vi "build group channel lists.vi"() -> ()   [LabVIEW 2018]
uses:
  <userlib>/_OpenG.lib/array/array.llb/Filter 1D Array (DBL)__ogtk.vi
  <userlib>/_OpenG.lib/array/array.llb/Remove Duplicates from 1D Array (DBL)__ogtk.vi
panel:
  out "negative card groups":T1(array[cluster])
  out "ACTIVE":dbl[](array[numeric])
  out "Groups":T1(array[cluster])
  out "Empty groups":T1(array[cluster])
  out "GROUP00":dbl[](array[numeric])
  out "TANK":dbl[](array[numeric])
  out "MRD":dbl[](array[numeric])
  out "VETO":dbl[](array[numeric])
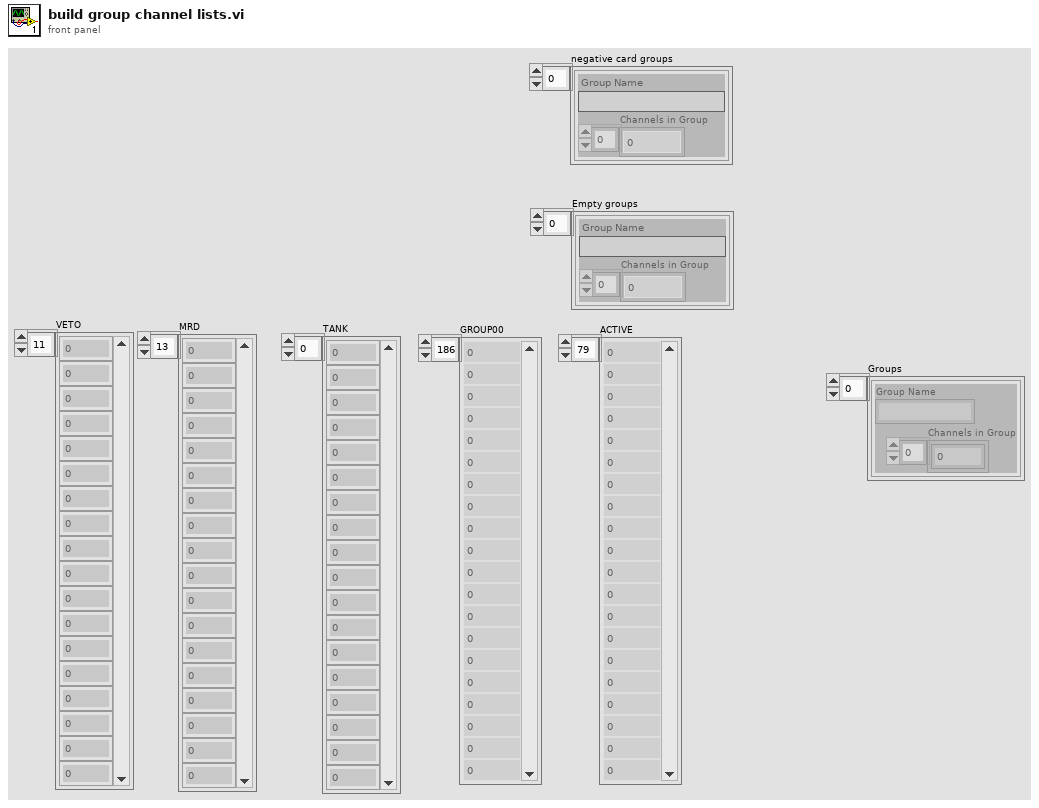
[diagram p1: front panel]
types:
  T1 = cluster{"Group Name":string, "Channels in Group":dbl[]}[]
  T2 = cluster{"Group Name":string, "Channels in Group":dbl[]}
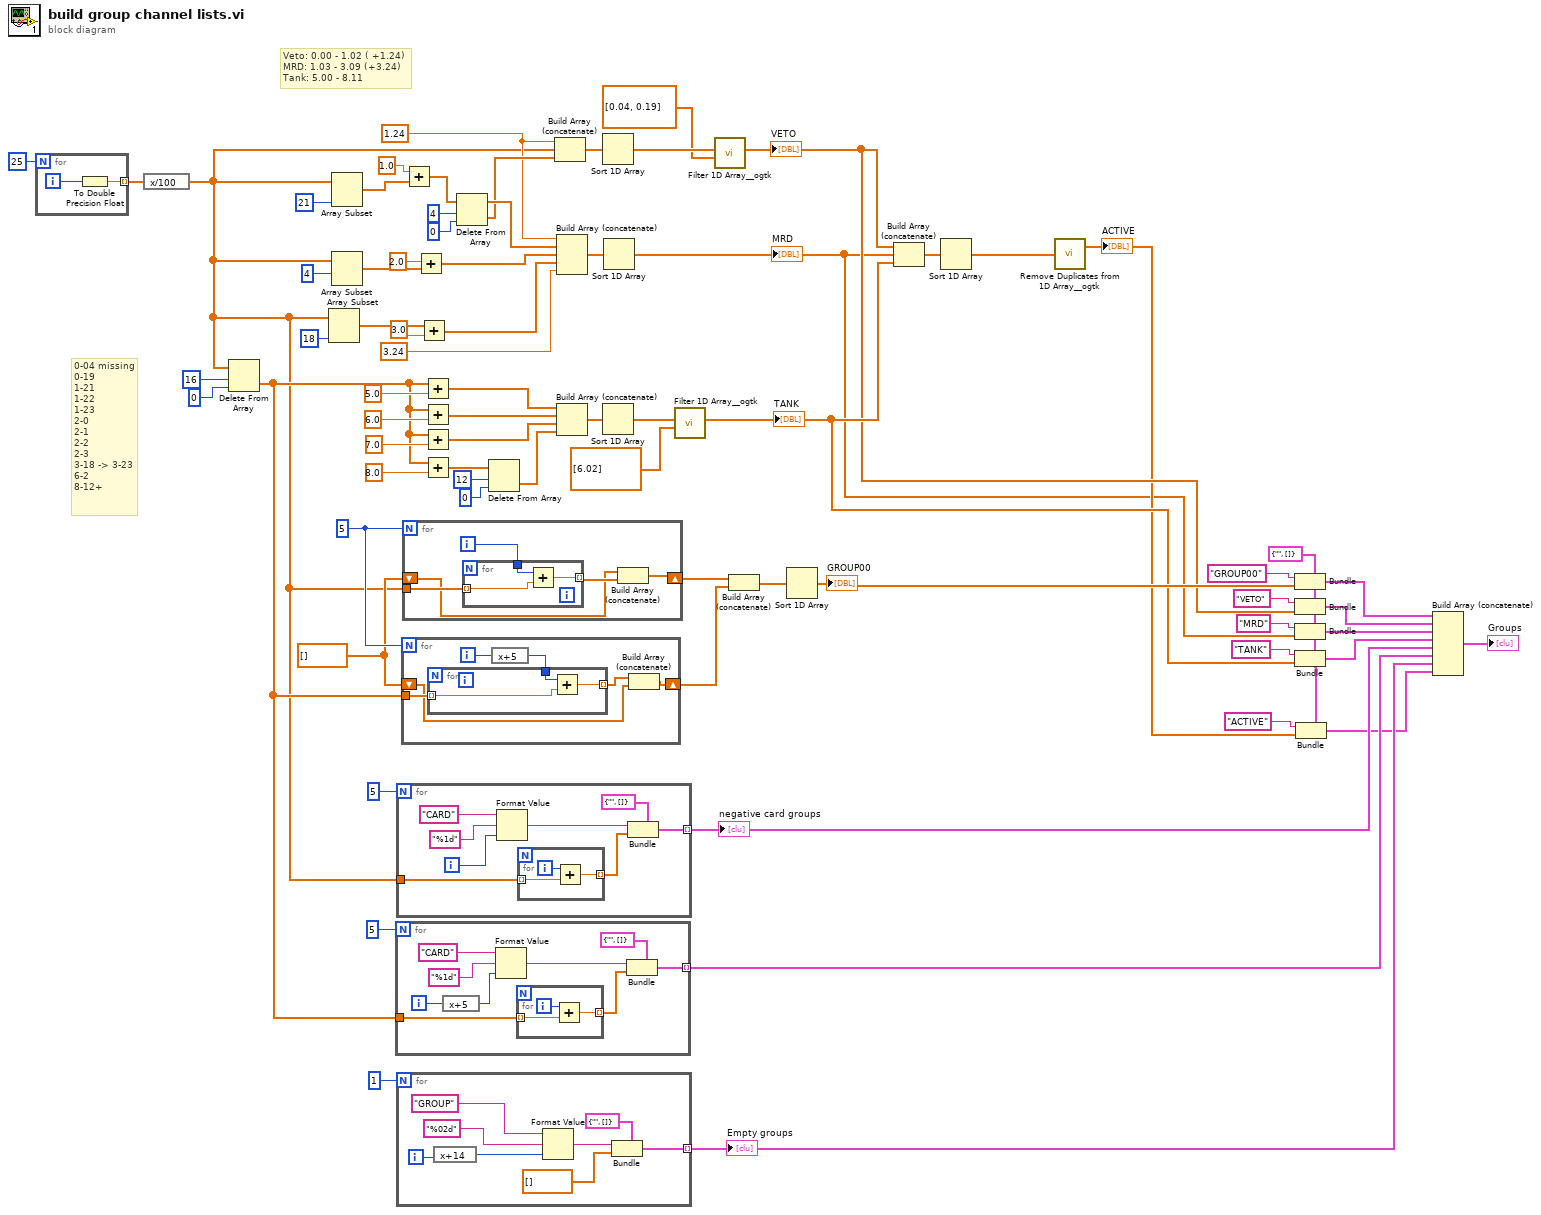
[diagram p0: block diagram]
diagram:
  w23 = T2 {"Group Name"="", "Channels in Group"=[]}
  w43 = dbl[] []
  w45 = 5
  w12 = 1.24 ("double precision float")
  # "0-04 missing\n0-19\n1-21\n1-22\n1-23\n2-0\n2-1\n2-2\n2-3\n3-18 -> 3-23\n6-2\n8-12+"
  # "Veto: 0.00 - 1.02 ( +1.24)\nMRD: 1.03 - 3.09 (+3.24)\nTank: 5.00 - 8.11"
  n1 = for {
    N: 25 -> [_]
    tunnel: [w73] -> w71 mode=indexing
    i -> [w74]
    n2 = To Double Precision Float(number=w74) -> (double precision float=w73:dbl)
  }
  n3 = expression code="x/100"(w71) -> (w8:dbl[])
  n4 = Delete From Array(array=w8, length=16, index=0) -> (deleted portion=w27:dbl[])  [unwired: 1 out]
  n5 = Array Subset(array=w8, length=18 ("index")) -> (w7:dbl[])  [unwired: 1 in]
  n6 = Array Subset(array=w8, length=21 ("index")) -> (w13:dbl[])  [unwired: 1 in]
  n7 = Array Subset(array=w8, index=4) -> (w11:dbl[])  [unwired: 1 in]
  n8 = for {
    N: 5 -> [_]
    tunnel: [w79] -> w25 mode=indexing
    tunnel: w27 -> [w78]
    i -> [w76]
    n9 = expression code="x+5"(w76) -> (w75:i32)
    n10 = Format Value(string ("")="CARD" ("Group Name"), format string="%1d" ("Group Name"), value (0)=w75) -> (output string=w80:string)
    n11 = for {
      tunnel: w78 -> [w85] mode=indexing
      tunnel: [w84] -> w77 mode=indexing
      i -> [w86]
      n12 = Add(x=w86, y=w85) -> (x+y=w84:dbl)
    }
    n13 = Bundle(cluster=T2 {"Group Name"="", "Channels in Group"=[]}, "Group Name"=w80, "Channels in Group"=w77) -> (w79:T2)
  }
  n14 = for {
    N: 5 -> [_]
    tunnel: [w90] -> w26 mode=indexing
    tunnel: w8 -> [w88]
    i -> [w89]
    n15 = Format Value(string ("")="CARD" ("Group Name"), format string="%1d" ("Group Name"), value (0)=w89) -> (output string=w91:string)
    n16 = for {
      tunnel: w88 -> [w96] mode=indexing
      tunnel: [w95] -> w87 mode=indexing
      i -> [w97]
      n17 = Add(x=w97, y=w96) -> (x+y=w95:dbl)
    }
    n18 = Bundle(cluster=T2 {"Group Name"="", "Channels in Group"=[]}, "Group Name"=w91, "Channels in Group"=w87) -> (w90:T2)
  }
  "negative card groups" <- w26
  n19 = for {
    N: 1 -> [_]
    tunnel: [w98] -> w24 mode=indexing
    i -> [w104]
    n20 = expression code="x+14"(w104) -> (w103:i32)
    n21 = Format Value(string ("")="GROUP" ("Group Name"), format string="%02d" ("Group Name"), value (0)=w103) -> (output string=w100:string)
    n22 = Bundle(cluster=T2 {"Group Name"="", "Channels in Group"=[]}, "Group Name"=w100, "Channels in Group"=dbl[] []) -> (w98:T2)
  }
  "Empty groups" <- w24
  n23 = for {
    N: w45 -> [_]
    tunnel: w27 -> [w111]
    shift-right: [w107] -> w42
    shift-left: w43 -> [w106]
    i -> [w110]
    n24 = expression code="x+5"(w110) -> (w109:i32)
    n25 = for {
      tunnel: w111 -> [w114] mode=indexing
      tunnel: [w113] -> w108 mode=indexing
      tunnel: w109 -> [w112]
      n26 = Add(x=w112, y=w114) -> (x+y=w113:dbl)
    }
    n27 = Build Array (concatenate)(w108, w106) -> (w107:dbl[])
  }
  n28 = for {
    N: w45 -> [_]
    tunnel: w8 -> [w119]
    shift-right: [w118] -> w44
    shift-left: w43 -> [w116]
    i -> [w115]
    n29 = for {
      tunnel: w119 -> [w122] mode=indexing
      tunnel: [w121] -> w117 mode=indexing
      tunnel: w115 -> [w120]
      n30 = Add(x=w120, y=w122) -> (x+y=w121:dbl)
    }
    n31 = Build Array (concatenate)(w116, w117) -> (w118:dbl[])
  }
  n32 = Add(x=1.0 ("double precision float"), y=w13) -> (x+y=w68:dbl[])
  n33 = Add(x=2.0 ("double precision float"), y=w11) -> (x+y=w64:dbl[])
  n34 = Add(x=w7, y=3.0 ("double precision float")) -> (x+y=w4:dbl[])
  n35 = Add(x=w27, y=5.0 ("double precision float")) -> (x+y=w53:dbl[])
  n36 = Add(x=w27, y=6.0 ("double precision float")) -> (x+y=w52:dbl[])
  n37 = Add(x=w27, y=7.0 ("double precision float")) -> (x+y=w51:dbl[])
  n38 = Add(x=w27, y=8.0 ("double precision float")) -> (x+y=w54:dbl[])
  n39 = Delete From Array(array=w68, length=4, index=0) -> (deleted portion=w63:dbl[], array with subset deleted=w65:dbl[])
  n40 = Delete From Array(array=w54, length=12, index=0) -> (deleted portion=w50:dbl[])  [unwired: 1 out]
  n41 = Build Array (concatenate)(w12, w8, w63) -> (w47:dbl[])
  n42 = Build Array (concatenate)(w12, w65, w64, w4, 3.24 ("double precision float")) -> (w48:dbl[])
  n43 = Build Array (concatenate)(w53, w52, w51, w50) -> (w49:dbl[])
  n44 = Sort 1D Array(array=w47) -> (sorted array=w17:dbl[])
  n45 = Sort 1D Array(array=w49) -> (sorted array=w19:dbl[])
  n46 = Sort 1D Array(array=w48) -> (sorted array=w2:dbl[])
  "MRD" <- w2
  n47 = call-poly <userlib>:"Filter 1D Array__ogtk.vi"("items to filter"=dbl[] [6.02], "array"=w19) -> ("filtered array"=w18:dbl[])  [unwired: 4 in, 1 out]
  "TANK" <- w18
  n48 = call-poly <userlib>:"Filter 1D Array__ogtk.vi"("items to filter"=dbl[] [0.04, 0.19], "array"=w17) -> ("filtered array"=w16:dbl[])  [unwired: 4 in, 1 out]
  "VETO" <- w16
  n49 = Build Array (concatenate)(w44, w42) -> (w46:dbl[])
  n50 = Sort 1D Array(array=w46) -> (sorted array=w31:dbl[])
  "GROUP00" <- w31
  n51 = Build Array (concatenate)(w16, w2, w18) -> (w21:dbl[])
  n52 = Sort 1D Array(array=w21) -> (sorted array=w1:dbl[])
  n53 = call-poly <userlib>:"Remove Duplicates from 1D Array__ogtk.vi"("Input Array"=w1) -> ("Output Array"=w14:dbl[])  [unwired: 1 out]
  "ACTIVE" <- w14
  n54 = Bundle(cluster=w23, "Group Name"="GROUP00", "Channels in Group"=w31) -> (w33:T2)
  n55 = Bundle(cluster=w23, "Group Name"="VETO", "Channels in Group"=w16) -> (w40:T2)
  n56 = Bundle(cluster=w23, "Group Name"="MRD", "Channels in Group"=w2) -> (w39:T2)
  n57 = Bundle(cluster=w23, "Group Name"="TANK", "Channels in Group"=w18) -> (w34:T2)
  n58 = Bundle(cluster=w23, "Group Name"="ACTIVE", "Channels in Group"=w14) -> (w22:T2)
  n59 = Build Array (concatenate)(w33, w40, w39, w34, w26, w25, w24, w22) -> (→"Groups":T1)
